vi "Read_DI_1_CVT.vi"() -> ()   [LabVIEW 2016]
uses:
  <vilib>/NI/Current Value Table/DataTypes/Boolean_Read.vi
  <vilib>/NI/Current Value Table/Type to Enum.vi
  <vilib>/NI/Current Value Table/DataTypes/Boolean_Type To Enum.vi
  <vilib>/Utility/file.llb/Read Delimited Spreadsheet (string).vi
  <vilib>/NI/Current Value Table/FGVs/CVT Globals.vi
  <vilib>/NI/Current Value Table/FGVs/Tag Memory.vi
  <vilib>/NI/Current Value Table/Memory Block.vi
  <vilib>/NI/Current Value Table/DataTypes/Boolean_Memory Block.vi
  <vilib>/NI/Current Value Table/Current Value Table.lvlib
panel:
  in  "stop":bool
  out "subarray 3":cluster{bool}[](array[cluster])
  out "subarray":cluster{bool}[](array[cluster])
  # "DOORS FB AND SENSOR\n                                  STATUS"
  # "Doctors Entrance Door-1 Open PB"
  # "Doctors Entrance Door-2 Open Proxy FB"
  # "Doctors Entrance Door-1 Open Inside PB"
  # "Main Entrance E-stop PB"
  # "Doctors Entrance Door-1 Open Proxy FB"
  # "Main Entrance-Strecther Entry PB"
  # "Doctors Entrance-Nose Mask Proxy"
  # "Main Entrance Door Open Inside PB"
  # "Doctors Entrance-Cap Proxy"
  # "Main Entrance Door Open Proxy FB"
  # "Doctors Entrance-Hand Sanitizer  Proxy"
  # "O.T Entrance-Nose Mask Proxy"
  # "Doctors Entrance Door-2 Open Inside PB"
  # "O.T. Entrance -Cap Proxy"
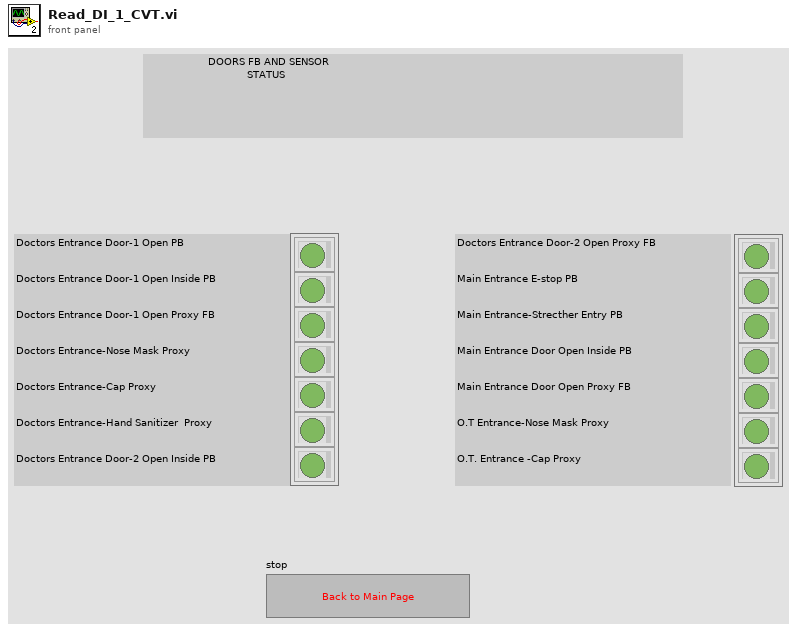
[diagram p1: front panel]
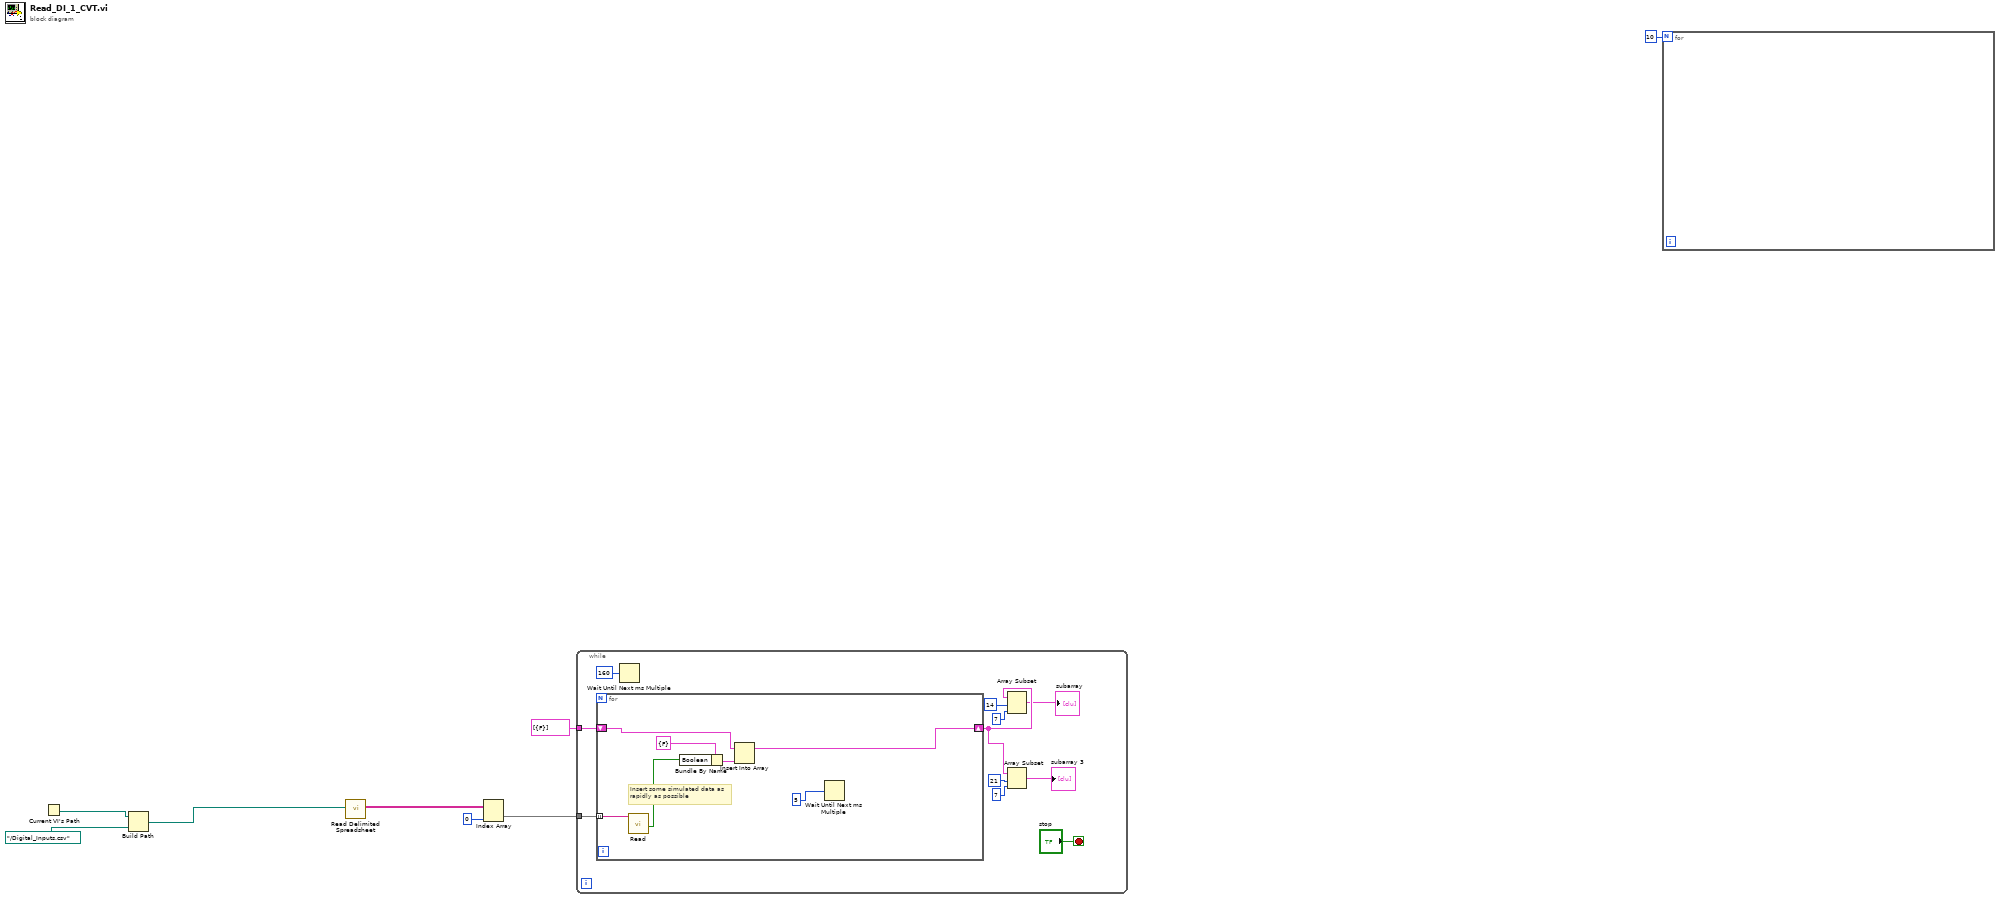
[diagram p0: block diagram]
diagram:
  n1 = Current VI's Path() -> (path=w3:path)
  n2 = Build Path(base path=w3, name or relative path=path "../Digital_Inputs.csv") -> (appended path=w1:path)
  n3 = call-poly <vilib>:"Read Delimited Spreadsheet.vi"("file path (dialog if empty)"=w1) -> ("all rows"=w6:string[][])  [unwired: 9 in, 5 out]
  n4 = Index Array "Index Array"(array=w6, index (col)=0 ("disabled index (col)")) -> (element=w4:string[])  [unwired: 1 in]
  n5 = while {
    tunnel: cluster{"Boolean":bool}[] [{"Boolean"=FALSE}] ("output array") -> [w19]
    tunnel: w4 -> [w18]
    stop <- "stop" stop-if-true
    n6 = for {
      shift-right: [w23] -> w14
      shift-left: w19 -> [w24]
      tunnel: w18 -> [w22] mode=indexing
      # "Insert some simulated data as\nrapidly as possible"
      n7 = call-poly <vilib>:"Read.vi"("Tag Name"=w22) -> ("Value"=w21:bool)  [unwired: 9 in, 1 out]
      n8 = Bundle By Name(cluster=cluster{"Boolean":bool} {"Boolean"=FALSE} ("Cluster"), "Boolean"=w21) -> (w25:cluster{"Boolean":bool})
      n9 = Insert Into Array(array=w24, new element=w25) -> (w23:cluster{"Boolean":bool}[])  [unwired: 1 in]
      n10 = Wait Until Next ms Multiple(millisecond multiple=u32 5 ("millisecond timer value")) -> ()  [unwired: 1 out]
    }
    n11 = Wait Until Next ms Multiple(millisecond multiple=u32 160 ("milliseconds to wait")) -> ()  [unwired: 1 out]
    n12 = Array Subset(array=w14, index=14, length=7) -> (→"subarray":cluster{"Boolean":bool}[])
    n13 = Array Subset "Array Subset"(array=w14, index=21, length=7) -> (→"subarray 3":cluster{"Boolean":bool}[])
  }
  n14 = for {
    N: 10 -> [_]
  }
